vi "stage-controller-globals.vi"() -> ()   [LabVIEW 2014]
uses:
  Stage SubVIs/ctts/small z increment.ctl
  Stage SubVIs/ctts/move stage.ctl
panel:
  out "Number of \nField Steps":dbl
  in  "Current Z":dbl
  in  "Current Y":dbl
  in  "Current X":dbl
  out "stage external trigger":refnum<user-event>
  in  "Field Step":u32=1 min=1 max=16
  in  "Field Size":enum16{"0", "1", "4", "9", "16"}(ring)=enum."16"
  out "YFieldDown":u32
  out "XFieldDiff":dbl
  out "YFieldUp":u32
  out "Previous\nsmall Z increment":T1
  out "Zmax":dbl
  out "Xmax":dbl
  out "Ymax":dbl
  out "Plot2":cluster{dbl[], dbl[]}={[101.064, 151.59599999999998], [100.915, 100.915]}
  out "Plot1":cluster{dbl[], dbl[]}={[101.064, 151.59599999999998], [50.457499999999996, 50.457499999999996]}
  out "Y mark down":dbl
  out "Y mark up":dbl
  out "X mark down":dbl
  out "X mark up":dbl
  # "************Not for interactive use************"
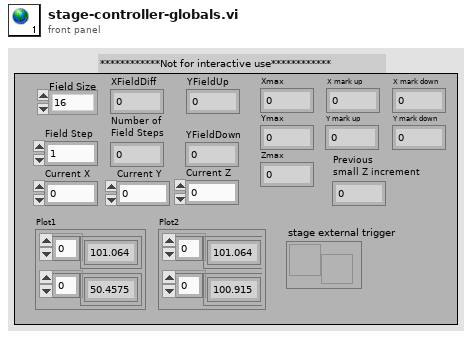
[diagram p1: front panel]
types:
  T1 = typedef "small z increment.ctl" = dbl
diagram:
